vi "FinalBrain.vi"() -> ()   [LabVIEW 2012]
uses:
  <vilib>/imath/engines/lvmath/Plug In/_Char/NIMS_CH_character datatype.ctl
  <vilib>/Utility/inputDevices.llb/closeKeyboard.vi
  <vilib>/Utility/inputDevices.llb/keyboardAcquire.vi
  <vilib>/imath/engines/lvmath2/RunTimeEngine/ErrorHandling/NIMS_Finalize Error.vi
  <vilib>/imath/engines/lvmath2/RunTimeEngine/Managers/WorkSpace/UID Generator.vi
  <vilib>/imath/engines/lvmath2/RunTimeEngine/Managers/SymbolTable/Clear UID.vi
  <vilib>/imath/engines/lvmath2/RunTimeEngine/NodeEndStatement/NIMS_NodeEndStatement_Output.vi
  <instcachedir>/0/NIMS_NodeEndStatement_Output_53EC0D466D134D7ABD903AC30B43404B.lvgen/NIMS_NodeEndStatement_Output_53EC0D466D134D7ABD903AC30B43404B_010.vi
  <instcachedir>/0/NIMS_NodeEndStatement_Output_53EC0D466D134D7ABD903AC30B43404B.lvgen/NIMS_NodeEndStatement_Output_53EC0D466D134D7ABD903AC30B43404B_012.vi
  <vilib>/imath/engines/lvmath2/RunTimeEngine/RunTimeType/NIMS_RunTimeType_From StrictType (excl LVString).vi
  <instcachedir>/0/NIMS_RunTimeType_From StrictType (excl LVString)_AC52D965D0864706932D20A05968E122.lvgen/NIMS_RunTimeType_From StrictType (excl LVString)_AC52D965D0864706932D20A05968E122_000.vi
  <vilib>/imath/engines/lvmath2/RunTimeEngine/LocalVariableDefStatement/MC_LocalVariableDefStatement_Display.vi
  <vilib>/imath/engines/lvmath2/RunTimeEngine/RunTimeType/NIMS_RunTimeType_Set Source Original Bool.vi
  <vilib>/imath/engines/lvmath/Plug In/_Char/NIMS_CH_Character RV to String.vi
  <instcachedir>/0/NIMS_NodeEndStatement_Output_53EC0D466D134D7ABD903AC30B43404B.lvgen/NIMS_NodeEndStatement_Output_53EC0D466D134D7ABD903AC30B43404B_009.vi
  <instcachedir>/0/NIMS_RunTimeType_From StrictType (excl LVString)_AC52D965D0864706932D20A05968E122.lvgen/NIMS_RunTimeType_From StrictType (excl LVString)_AC52D965D0864706932D20A05968E122_001.vi
  <vilib>/imath/engines/lvmath2/RunTimeEngine/Managers/SymbolTable/NIMS_WorkSpace.lvlib
panel:
  out "BS Timed Out":bool
  out "Base Station":string
  in  "error in (no error)":errorcluster
  in  "Tab Control":T1(tab)
  in  "Read Color":bool
  out "Bump Sensor 2":bool
  out "Distance 2, CM":dbl
  out "IR Volts Nav":dbl
  out "Red":dbl(knob) scale=0.0..100.0
  out "Green":dbl(knob) scale=0.0..100.0
  out "Blue":dbl(knob) scale=0.0..100.0
  out "Color Chosen":u32(colorbox)
  out "Bump Sensor 1":bool
  out "IR Volts Align":dbl
  out "Distance 1, CM":dbl
  in  "stop":bool
  out "Left Arm":i32
  out "Right Arm":i32
  in  "Arm":i32(slide)=1500 scale=500.0..2500.0
  out "Port\nMotor":i32
  out "Starboard\nMotor":i32
  out "Port Speed":i32(knob) scale=1000.0..2000.0
  out "Starboard Speed":i32(knob) scale=1000.0..2000.0
  out "Speed Balance":i32(knob) scale=-600.0..600.0
  in  "Initiate Mission":bool
  out "Angle to Target":i32
  out "Distance to Target":i32
  out "Bump 2":bool
  out "Bump  1":bool
  out "Current Target":i32
  out "Obstacle Detected":bool
  out "Primitive Engaged":string
  out "Desired Heading":i32
  out "Target Y":i32
  out "Target X":i32
  out "Current Y":i32
  out "Current X":i32
  out "Current Heading":i32
  out "Target Locations":i32[][](array[numeric])
  in  "Step Size":i32=5
  in  "PC Status":i32=1
  out "String Received":string
  out "return count":u32
  out "bytes written":u32
  out "Blinky":bool
  in  "String":string="$CS1500P1500R1500L1500P1500H   1\n"
  in  "FULLSTOP":bool
  in  "VISA resource name":refnum<visa-resource-name>="COM7"
  # "ROBOT CONTROL VI\nSoftware Phase for Autonomy\n\nVPreston\n4/14/2014"
  # "Thought:\n- Need to calibrate the accelerometer each time, which means that the first step will need to be \nSpinning in place at a set location (likely the landing zone)\n- Is this worth it?  If not, a simple heading can be developed based upon movement from the \ncamera, though this is likely to be glitchy and less reliable....\n\n- Calculate heading with accelerometer in the hindbrain, pass this up to PC\nOR\n- Calculate heading from base station in PC"
  # "Use this tab to make sure your sensors are happy and working properly."
  # "Motor Control"
  # "Direction of thrust"
  # "Purple Target - 80, 230\nYellow Target - \nRed Target - 37, 78 \nGreen Target - 258, 43 \nBlue Target - 492, 63"
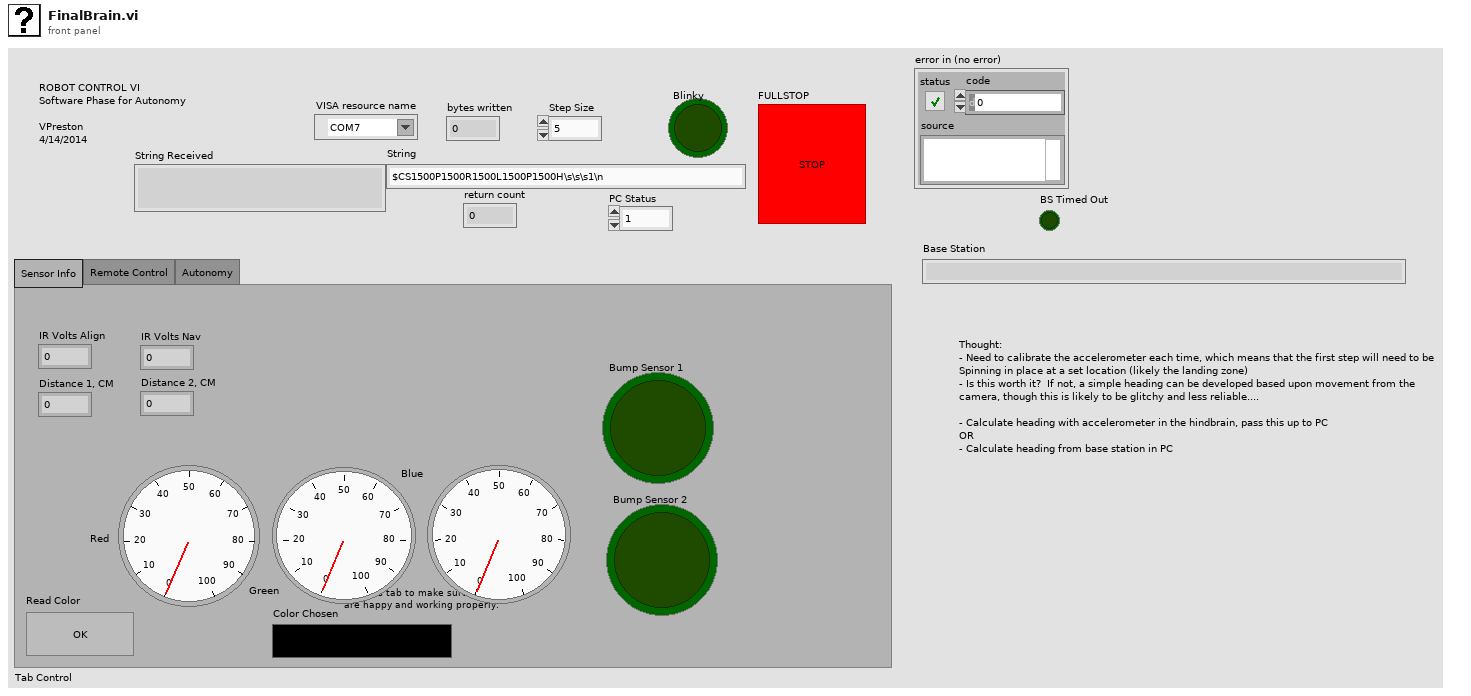
[diagram p1: front panel]
types:
  T1 = enum32{"Sensor Info", "Remote Control", "Autonomy"}
  T2 = enum16{"0", "1", "2", "3", "4", "5", "6", "7", "8", "9", "A", "B", "C", "D", "E", "F", "G", "H", "I", "J", "K", "L", "M", "N", "O", "P", "Q", "R", "S", "T", "U", "V", "W", "X", "Y", "Z", "F1", "F2", "F3", "F4", "F5", "F6", "F7", "F8", "F9", "F10", "F11", "F12", "F13", "F14", "F15", "ADD", "BACK", "BACKSLASH", "CAPITAL", "COMMA", "DECIMAL", "DELETE", "DIVIDE", "DOWN", "END", "EQUALS", "ESCAPE", "GRAVE (`)", "HOME", "INSERT", "LBRACKET", "LCONTROL", "LEFT", "L ALT", "LSHIFT", "LWIN", "MINUS", "MULTIPLY", "NEXT", "NUMLOCK", "NUMPAD_0", "NUMPAD_1", "NUMPAD_2", "NUMPAD_3", "NUMPAD_4", "NUMPAD_5", "NUMPAD_6", "NUMPAD_7", "NUMPAD_8", "NUMPAD_9", "PAUSE", "PERIOD", "PRIOR (PG UP)", "RBRACKET", "RCONTROL", "RETURN", "RIGHT", "R ALT", "RSHIFT", "RWIN", "SCROLL", "SEMICOLON", "SLASH", "SPACE", "SUBTRACT", "TAB", "UP", "ENTER (num pad)", "' (quote)"}[]
  T3 = enum16{"0", "1", "2", "3", "4", "5", "6", "7", "8", "9", "A", "B", "C", "D", "E", "F", "G", "H", "I", "J", "K", "L", "M", "N", "O", "P", "Q", "R", "S", "T", "U", "V", "W", "X", "Y", "Z", "F1", "F2", "F3", "F4", "F5", "F6", "F7", "F8", "F9", "F10", "F11", "F12", "F13", "F14", "F15", "ADD", "BACK", "BACKSLASH", "CAPITAL", "COMMA", "DECIMAL", "DELETE", "DIVIDE", "DOWN", "END", "EQUALS", "ESCAPE", "GRAVE (`)", "HOME", "INSERT", "LBRACKET", "LCONTROL", "LEFT", "L ALT", "LSHIFT", "LWIN", "MINUS", "MULTIPLY", "NEXT", "NUMLOCK", "NUMPAD_0", "NUMPAD_1", "NUMPAD_2", "NUMPAD_3", "NUMPAD_4", "NUMPAD_5", "NUMPAD_6", "NUMPAD_7", "NUMPAD_8", "NUMPAD_9", "PAUSE", "PERIOD", "PRIOR (PG UP)", "RBRACKET", "RCONTROL", "RETURN", "RIGHT", "R ALT", "RSHIFT", "RWIN", "SCROLL", "SEMICOLON", "SLASH", "SPACE", "SUBTRACT", "TAB", "UP", "ENTER (num pad)", "' (quote)"}
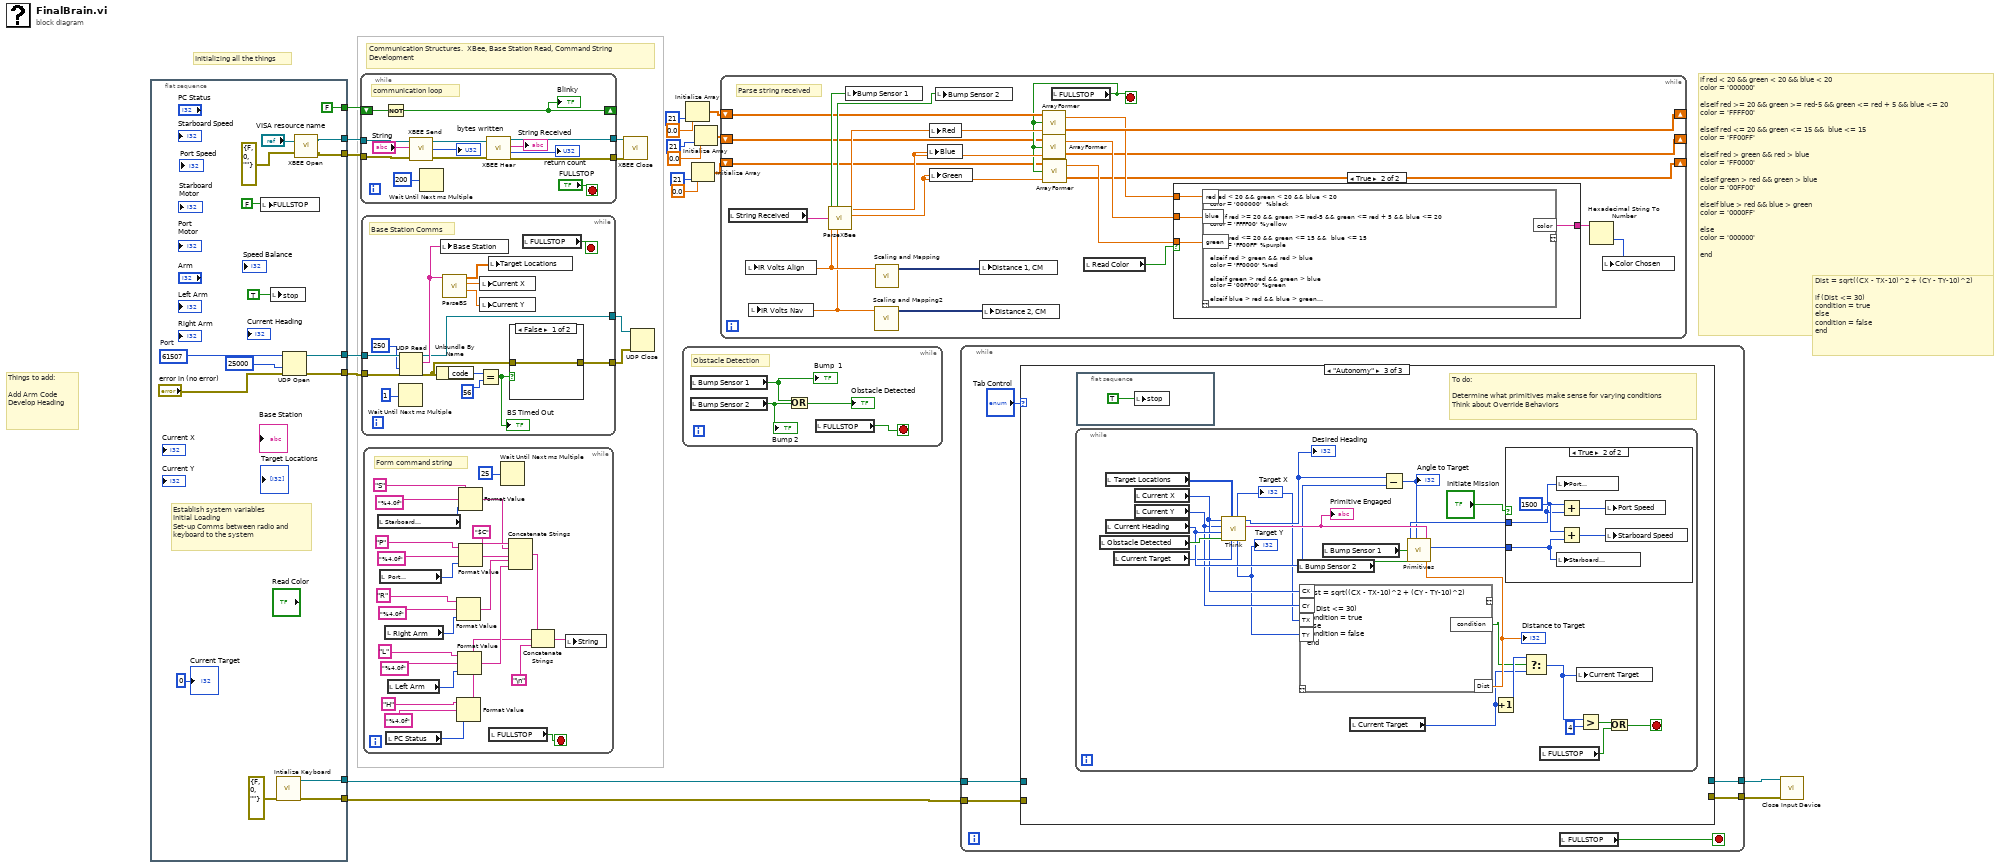
[diagram p0: block diagram]
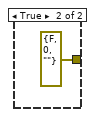
[diagram p2: hidden frame]
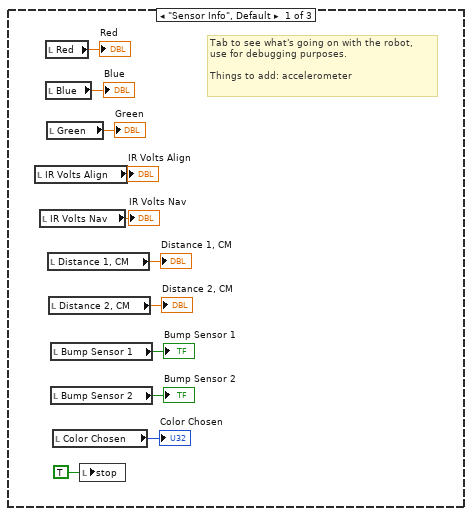
[diagram p3: hidden frame]
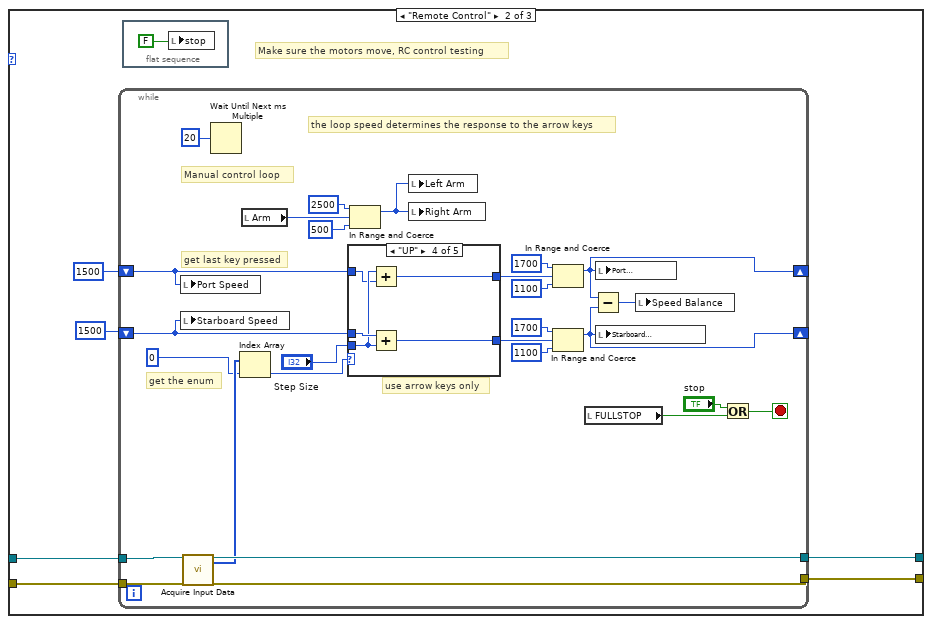
[diagram p4: hidden frame]
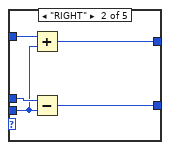
[diagram p6: hidden frame]
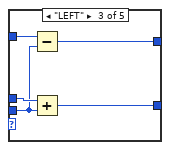
[diagram p7: hidden frame]
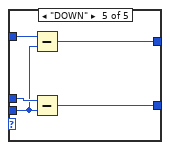
[diagram p8: hidden frame]
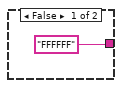
[diagram p10: hidden frame]
diagram:
  # "Dist = sqrt((CX - TX-10)^2 + (CY - TY-10)^2)\n\nif (Dist <= 30)\ncondition = true\nelse\ncondition = false\nend"
  # "if red < 20 && green < 20 && blue < 20\ncolor = '000000'\n\nelseif red >= 20 && green >= red-5 && green <= red + 5 && blue <= 20\ncolor = 'FFFF00'\n\nelseif red <= 20 && green <= 15 &&  blue <= 15\ncolor = 'FF00FF'\n\nelseif red > green && red > blue\ncolor = 'FF0000'\n\nelseif green > red && green > blue\ncolor = '00FF00'\n\nelseif blue > red && blue > green\ncolor = '0000FF' \n\nelse\ncolor = '000000'\n\nend"
  # "Initializing all the things"
  # "Communication Structures.  XBee, Base Station Read, Command String Development"
  # "Things to add: \n\nAdd Arm Code\nDevelop Heading"
  n1 = flat-sequence {
    tunnel: [w38] -> w22
    tunnel: [w26] -> w21
    tunnel: [FALSE] -> w18
    tunnel: [w33] -> w17
    tunnel: [w32] -> w16
    tunnel: [w25] -> w10
    tunnel: [w27] -> w13
    frame #0 {
      w29 = u16 61507  # Port
      # "Establish system variables\nInitial Loading\nSet-up Comms between radio and\nkeyboard to the system"
      n2 = local write "FULLSTOP"(FALSE) -> ()
      n3 = local write "stop"(TRUE) -> ()
      n4 = call <vilib>:"Intialize Keyboard.vi"("error in (no error)"=errorcluster {"status"=FALSE, "code"=0, "source"=""}) -> ("error out"=w32:errorcluster, "device ID"=w33:refnum<k1>)  [unwired: 9 in]
      n5 = UDP Open(8:"error in (no error)", 9:25000 ("timeout ms (25000)"), 11:w29) -> (port=w25:refnum<k16>, 0:w27:errorcluster)  [unwired: 2 in, 1 out]
      n6 = call "XBEE Open.vi"("error in"=errorcluster {"status"=FALSE, "code"=0, "source"=""}, "VISA resource name"="VISA resource name") -> ("error out"=w26:errorcluster, "VISA resource name out"=w38:refnum<visa-resource-name>)
      "Current Target" <- 0
    }
  }
  n7 = while {
    tunnel: w22 -> [w51]
    tunnel: w21 -> [w50]
    tunnel: [w45] -> w20
    tunnel: [w44] -> w19
    shift-right: [w48] -> _
    shift-left: w18 -> [w49]
    stop <- "FULLSTOP" stop-if-true
    # "communication loop"
    n8 = Not(x=w49) -> (.not. x?=w48:bool)
    "Blinky" <- w48
    n9 = call "XBEE Send.vi"("error in (no error)"=w50, "String"="String", "VISA resource name"=w51) -> ("error out"=w41:errorcluster, "return count"=→"bytes written":u32, "VISA resource name out"=w42:refnum<visa-resource-name>)
    n10 = Wait Until Next ms Multiple(millisecond multiple=u32 200) -> ()  [unwired: 1 out]
    n11 = call "XBEE Hear.vi"("VISA resource name"=w42, "error in (no error)"=w41) -> ("VISA resource name out"=w45:refnum<visa-resource-name>, "String Received"=→"String Received":string, "return count"=→"return count":u32, "error out"=w44:errorcluster)
  }
  n12 = while {
    tunnel: w10 -> [w67]
    tunnel: w13 -> [w66]
    tunnel: [w54] -> w12
    tunnel: [w53] -> w11
    stop <- w59 stop-if-true
    # "Base Station Comms"
    n13 = Wait Until Next ms Multiple(millisecond multiple=u32 1) -> ()  [unwired: 1 out]
    n14 = UDP Read(connection ID=w67, timeout ms (25000)=250, 8:w66) -> (data out=w58:string, error out=w62:errorcluster, 3:w54:refnum<k16>)  [unwired: 1 in, 2 out]
    n15 = Unbundle By Name(w62) -> ("code"=w61:i32)
    n16 = local write "Base Station"(w58) -> ()
    n17 = call "ParseBS.vi"("BS String"=w58) -> ("Y Pos"=w55:dbl, "X Pos"=w56:dbl, "Target Locations"=w57:dbl[][])  [unwired: 8 in]
    n18 = Equal?(x=w61, y=56) -> (x = y?=w60:bool)
    "BS Timed Out" <- w60
    n19 = local write "Current X"(w56) -> ()
    n20 = local write "Current Y"(w55) -> ()
    n21 = local write "Target Locations"(w57) -> ()
    n22 = case shown="False" w60 {
      tunnel: [w68 errorcluster {"status"=FALSE, "code"=0, "source"=""} ("error out")] -> w53
      tunnel: w62 -> [w68 _]
      frame False {
      }
      frame True {
      }
    }
    n23 = local read "FULLSTOP"() -> (w59:bool)
  }
  n24 = while {
    stop <- w95 stop-if-true
    # "Form command string"
    n25 = local read "Starboard\nMotor"() -> (w92:i32)
    n26 = local read "Port\nMotor"() -> (w89:i32)
    n27 = local read "Right Arm"() -> (w83:i32)
    n28 = local read "PC Status"() -> (w74:i32)
    n29 = local read "Left Arm"() -> (w80:i32)
    n30 = Format Value(string ("")="R", format string="%4.0f", value (0)=w83) -> (output string=w79:string)
    n31 = Format Value(string ("")="H", format string="%4.0f", value (0)=w74) -> (output string=w71:string)
    n32 = Format Value(string ("")="L", format string="%4.0f", value (0)=w80) -> (output string=w78:string)
    n33 = Format Value(string ("")="S", format string="%4.0f", value (0)=w92) -> (output string=w87:string)
    n34 = Format Value(string ("")="P", format string="%4.0f", value (0)=w89) -> (output string=w86:string)
    n35 = local read "FULLSTOP"() -> (w95:bool)
    n36 = Wait Until Next ms Multiple(millisecond multiple=u32 25) -> ()  [unwired: 1 out]
    n37 = Concatenate Strings("$C", w87, w86, w79, w78) -> (w73:string)
    n38 = Concatenate Strings(w73, w71, "\n") -> (w77:string)
    n39 = local write "String"(w77) -> ()
  }
  n40 = call "XBEE Close.vi"("error in (no error)"=w19, "VISA resource name"=w20) -> ()
  n41 = UDP Close(connection ID=w12, 8:w11) -> ()  [unwired: 2 out]
  n42 = while {
    stop <- w99 stop-if-true
    # "Obstacle Detection"
    n43 = local read "Bump Sensor 1"() -> (w98:bool)
    "Bump  1" <- w98
    n44 = local read "Bump Sensor 2"() -> (w97:bool)
    "Bump 2" <- w97
    n45 = Or(x=w98, y=w97) -> (x .or. y?=→"Obstacle Detected":bool)
    n46 = local read "FULLSTOP"() -> (w99:bool)
  }
  n47 = Initialize Array(0.0 ("element"), 21 ("dimension size")) -> (w9:dbl[])
  n48 = Initialize Array(0.0 ("element"), 21 ("dimension size")) -> (w1:dbl[])
  n49 = Initialize Array(0.0 ("element"), 21 ("dimension size")) -> (w2:dbl[])
  n50 = while {
    shift-right: [w111] -> _
    shift-left: w9 -> [w112]
    shift-right: [w103] -> _
    shift-left: w2 -> [w104]
    shift-right: [w101] -> _
    shift-left: w1 -> [w102]
    stop <- w105 stop-if-true
    # "Parse string received"
    n51 = local read "String Received"() -> (w118:string)
    n52 = call "ParseXBee.vi"("XBee String"=w118) -> ("Bump 1"=w117:bool, "Bump 2"=w116:bool, "IR Align"=w115:dbl, "IR Nav"=w114:dbl, "Red"=w113:dbl, "Blue"=w109:dbl, "Green"=w107:dbl)  [unwired: 3 in]
    n53 = local write "IR Volts Align"(w115) -> ()
    n54 = local write "IR Volts Nav"(w114) -> ()
    n55 = local write "Bump Sensor 1"(w117) -> ()
    n56 = call "Scaling and Mapping2"("Signals"=w114) -> ("Scaled Signals"=w119:dynamicdata)  [unwired: 9 in, 1 out]
    n57 = call "Scaling and Mapping"("Signals"=w115) -> ("Scaled Signals"=w120:dynamicdata)  [unwired: 9 in, 1 out]
    n58 = local write "Blue"(w109) -> ()
    n59 = local write "Red"(w113) -> ()
    n60 = local write "Green"(w107) -> ()
    n61 = local write "Bump Sensor 2"(w116) -> ()
    n62 = local write "Distance 1, CM"(w120) -> ()
    n63 = local write "Distance 2, CM"(w119) -> ()
    n64 = local read "FULLSTOP"() -> (w105:bool)
    n65 = call "ArrayFormer.vi"("New Data"=w113, "stop"=w105, "Existing"=w112) -> ("Current"=w111:dbl[], "Average"=w110:dbl)
    n66 = call "ArrayFormer.vi"("New Data"=w109, "stop"=w105, "Existing"=w104) -> ("Current"=w103:dbl[], "Average"=w108:dbl)
    n67 = call "ArrayFormer.vi"("New Data"=w107, "stop"=w105, "Existing"=w102) -> ("Current"=w101:dbl[], "Average"=w106:dbl)
    n68 = local read "Read Color"() -> (w100:bool)
    n69 = case shown="True" w100 {
      tunnel: ["FFFFFF" w127] -> w122
      tunnel: w110 -> [_ w126]
      tunnel: w108 -> [_ w125]
      tunnel: w106 -> [_ w124]
      frame False {
      }
      frame True {
        n70 = mathscript code="if red < 20 && green < 20 && blue < 20\ncolor = '000000'  %black\n\nelseif red >= 20 && green >= red-5 && green <= red + 5 && blue <= 20\ncolor = 'FFFF00' %yellow\n\nelseif red <= 20 && green <= 15 &&  blue <= 15\ncolor = 'FF00FF' %purple\n\nelseif red > green && red > blue\ncolor = 'FF0000' %red\n\nelseif green > red && green > blue\ncolor = '00FF00' %green\n\nelseif blue > red && blue > green\ncolor = '0000FF' %blue\n\nelse\ncolor = '000000'\n\nend"("red"=w126, "blue"=w125, "green"=w124) -> ("color"=w127:string)  [unwired: 1 in, 1 out]
      }
    }
    n71 = Hexadecimal String To Number(string=w122) -> (number=w121:u32)  [unwired: 2 in, 1 out]
    n72 = local write "Color Chosen"(w121) -> ()
  }
  n73 = while {
    tunnel: w17 -> [w418]
    tunnel: w16 -> [w417]
    tunnel: [w416] -> w15
    tunnel: [w415] -> w14
    stop <- w414 stop-if-true
    n74 = case shown="\"Autonomy\"" "Tab Control" {
      tunnel: w418 -> [_ w436 _]
      tunnel: w417 -> [_ w435 _]
      tunnel: [_ w432 _] -> w416
      tunnel: [_ w431 _] -> w415
      frame "Sensor Info", Default {
        # "Tab to see what's going on with the robot, \nuse for debugging purposes.  \n\nThings to add: accelerometer"
        n75 = local read "IR Volts Align"() -> (→"IR Volts Align":dbl)
        n76 = local read "IR Volts Nav"() -> (→"IR Volts Nav":dbl)
        n77 = local read "Red"() -> (→"Red":dbl)
        n78 = local read "Blue"() -> (→"Blue":dbl)
        n79 = local read "Green"() -> (→"Green":dbl)
        n80 = local read "Distance 1, CM"() -> (→"Distance 1, CM":dbl)
        n81 = local read "Distance 2, CM"() -> (→"Distance 2, CM":dbl)
        n82 = local read "Bump Sensor 1"() -> (→"Bump Sensor 1":bool)
        n83 = local read "Bump Sensor 2"() -> (→"Bump Sensor 2":bool)
        n84 = local read "Color Chosen"() -> (→"Color Chosen":u32)
        n85 = local write "stop"(TRUE) -> ()
      }
      frame "Remote Control" {
        # "Make sure the motors move, RC control testing"
        n86 = while {
          tunnel: [w464] -> w431
          tunnel: [w463] -> w432
          shift-right: [w447] -> _
          shift-left: 1500 -> [w449]
          shift-right: [w446] -> _
          shift-left: 1500 -> [w448]
          tunnel: w436 -> [w439]
          tunnel: w435 -> [w438]
          stop <- w440 stop-if-true
          # "use arrow keys only"
          # "Manual control loop"
          # "get the enum"
          # "the loop speed determines the response to the arrow keys"
          # "get last key pressed"
          n87 = local write "Port Speed"(w448) -> ()
          n88 = local write "Starboard Speed"(w449) -> ()
          n89 = call-poly <vilib>:"Acquire Input Data.vi"("device ID"=w439, "error in (no error)"=w438) -> ("device ID"=w463:refnum<k1>, "keys pressed"=w462:T2, "error out"=w464:errorcluster)  [unwired: 15 in]
          n90 = Wait Until Next ms Multiple(millisecond multiple=u32 20) -> ()  [unwired: 1 out]
          n91 = Index Array(array=w462, index=0) -> (element=w460:T3)
          n92 = local read "Arm"() -> (w444:i32)
          n93 = case shown="\"UP\"" w460 {
            tunnel: w449 -> [w466 w468 w473 w481 w486]
            tunnel: [w466 w469 w474 w480 w485] -> w458
            tunnel: w448 -> [w465 w471 w475 w478 w484]
            tunnel: [w465 w470 w476 w477 w482] -> w450
            tunnel: "Step Size" -> [_ w467 w472 w479 w483]
            frame "0", Default {
            }
            frame "RIGHT" {
              n94 = Add(x=w471, y=w467) -> (x+y=w470:i32)
              n95 = Subtract(x=w468, y=w467) -> (x-y=w469:i32)
            }
            frame "LEFT" {
              n96 = Subtract(x=w475, y=w472) -> (x-y=w476:i32)
              n97 = Add(x=w473, y=w472) -> (x+y=w474:i32)
            }
            frame "UP" {
              n98 = Add(x=w479, y=w478) -> (x+y=w477:i32)
              n99 = Add(x=w481, y=w479) -> (x+y=w480:i32)
            }
            frame "DOWN" {
              n100 = Subtract(x=w484, y=w483) -> (x-y=w482:i32)
              n101 = Subtract(x=w486, y=w483) -> (x-y=w485:i32)
            }
          }
          n102 = In Range and Coerce(upper limit=2500, x=w444, lower limit=500) -> (coerced(x)=w443:i32)  [unwired: 1 out]
          n103 = local write "Left Arm"(w443) -> ()
          n104 = local write "Right Arm"(w443) -> ()
          n105 = In Range and Coerce(upper limit=1700, x=w450, lower limit=1100) -> (coerced(x)=w446:i32)  [unwired: 1 out]
          n106 = In Range and Coerce(upper limit=1700, x=w458, lower limit=1100) -> (coerced(x)=w447:i32)  [unwired: 1 out]
          n107 = local read "FULLSTOP"() -> (w441:bool)
          n108 = Subtract(x=w446, y=w447) -> (x-y=w445:i32)
          n109 = local write "Port\nMotor"(w446) -> ()
          n110 = local write "Starboard\nMotor"(w447) -> ()
          n111 = local write "Speed Balance"(w445) -> ()
          n112 = Or(x="stop", y=w441) -> (x .or. y?=w440:bool)
        }
        n113 = flat-sequence {
          frame #0 {
            n114 = local write "stop"(FALSE) -> ()
          }
        }
      }
      frame "Autonomy" {
        # "To do:\n\nDetermine what primitives make sense for varying conditions\nThink about Override Behaviors"
        n115 = while {
          stop <- w494 stop-if-true
          n116 = local read "Obstacle Detected"() -> (w510:bool)
          n117 = local read "Target Locations"() -> (w511:i32[][])
          n118 = local read "Current Heading"() -> (w505:i32)
          n119 = local read "Current Target"() -> (w502:i32)
          n120 = local read "Current X"() -> (w500:i32)
          n121 = local read "Current Y"() -> (w499:i32)
          n122 = call "Think.vi"("Target"=w502, "Target Locations"=w511, "Override Engaged"=w510, "Current Heading"=w505, "Y Position"=w499, "X Position"=w500) -> ("Executable Primitive"=w509:string, "Desired Heading"=w506:i32, "Desired Y"=w497:i32, "Desired X"=w498:i32)  [unwired: 2 in]
          "Target Y" <- w497
          "Desired Heading" <- w506
          "Primitive Engaged" <- w509
          "Target X" <- w498
          n123 = local read "Bump Sensor 2"() -> (w507:bool)
          n124 = mathscript code="Dist = sqrt((CX - TX-10)^2 + (CY - TY-10)^2)\n\nif (Dist <= 30)\ncondition = true\nelse\ncondition = false\nend"("CX"=w500, "CY"=w499, "TX"=w498, "TY"=w497) -> ("Dist"=w492:cdb, "condition"=w489:bool)  [unwired: 1 in, 1 out]
          "Distance to Target" <- w492
          n125 = local read "Bump Sensor 1"() -> (w508:bool)
          n126 = local read "Current Target"() -> (w490:i32)
          n127 = Subtract(x=w506, y=w505) -> (x-y=w493:i32)
          "Angle to Target" <- w493
          n128 = call "Primitives.vi"("Angle to Target"=w493, "Bump 1"=w508, "Bump 2"=w507, "Primitive"=w509, "Distance to Target"=w492) -> ("Port Speed"=w503:i32, "Starboard Speed"=w504:i32)  [unwired: 2 in]
          n129 = Increment(x=w490) -> (x+1=w491:i32)
          n130 = case shown="True" "Initiate Mission" {
            tunnel: w504 -> [_ w516]
            tunnel: w503 -> [_ w513]
            frame False {
            }
            frame True {
              w514 = 1500
              n131 = local write "Port\nMotor"(w513) -> ()
              n132 = local write "Starboard\nMotor"(w516) -> ()
              n133 = Add(x=w514, y=w513) -> (x+y=w512:i32)
              n134 = Add(x=w514, y=w516) -> (x+y=w515:i32)
              n135 = local write "Port Speed"(w512) -> ()
              n136 = local write "Starboard Speed"(w515) -> ()
            }
          }
          n137 = Select(t=w491, s=w489, f=w490) -> (s? t:f=w488:i32)
          n138 = local read "FULLSTOP"() -> (w495:bool)
          n139 = local write "Current Target"(w488) -> ()
          n140 = Greater?(x=w488, y=4) -> (0:w496:bool)
          n141 = Or(x=w496, y=w495) -> (x .or. y?=w494:bool)
        }
        n142 = flat-sequence {
          frame #0 {
            n143 = local write "stop"(TRUE) -> ()
          }
        }
      }
    }
    n144 = local read "FULLSTOP"() -> (w414:bool)
  }
  n145 = call-poly <vilib>:"Close Input Device.vi"("error in (no error)"=w14, "device ID"=w15) -> ()  [unwired: 8 in, 1 out]
